vi "Data Format.vi"(9 "Table":refnum<vi>) -> (0 "title":string[](array[string]), 2 "Data":string[](array[string]))   [LabVIEW 2017]
panel:
  out "Error_Description":string
  out "Table":string[][](array[string])
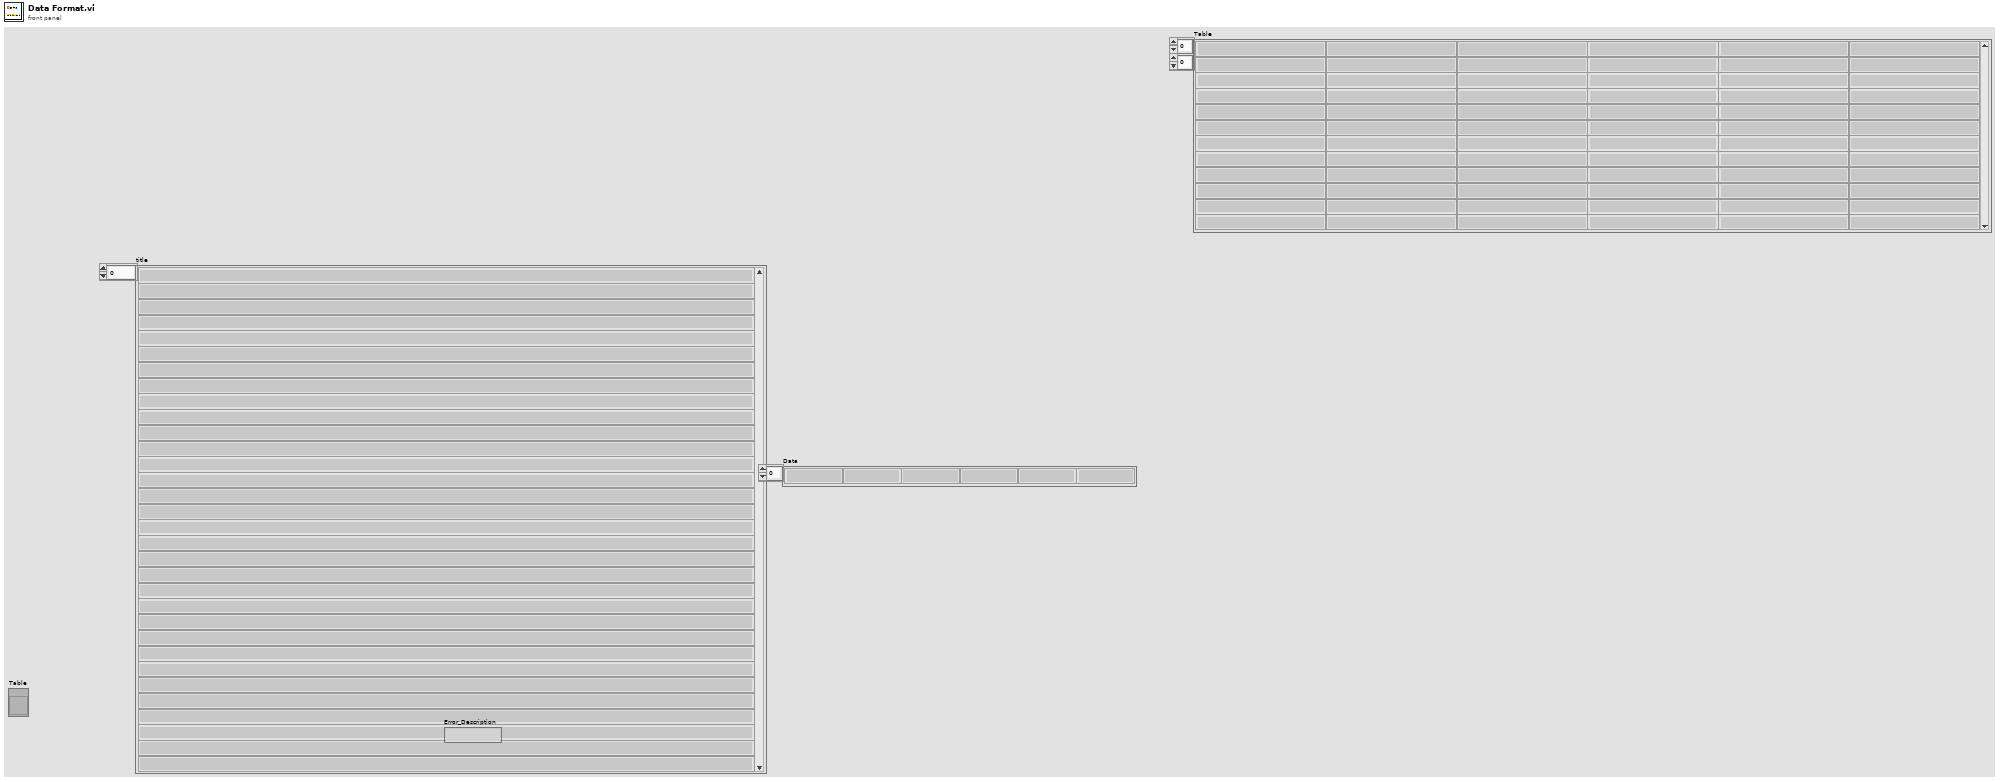
[diagram p1: front panel]
types:
  T1 = typedef "HD Config.ctl" = cluster{" PC":cluster{"PC Address":u8[], "PC Port":i32}, "FCO":cluster{"COM":refnum<visa-resource-name>, "Baudrate":u32}, "DC Power ":cluster{"COM":refnum<visa-resource-name>, "Baudrate":u32}, "PW3336":cluster{"COM":refnum<visa-resource-name>, "Baudrate":u32}, "Lefoo":cluster{"COM":refnum<visa-resource-name>, "Baudrate":u32}, "Tempt&Hum":cluster{"COM":refnum<visa-resource-name>, "Baudrate":u32}, "DIPC":cluster{"COM":refnum<visa-resource-name>}, "Daemon":cluster{"IP Address":string, "Port":u16, "Retry":u16}, "URAT":cluster{"COM":refnum<visa-resource-name>, "Baudrate":u32}, "Fail_resume_mode":bool, "GRR":bool}
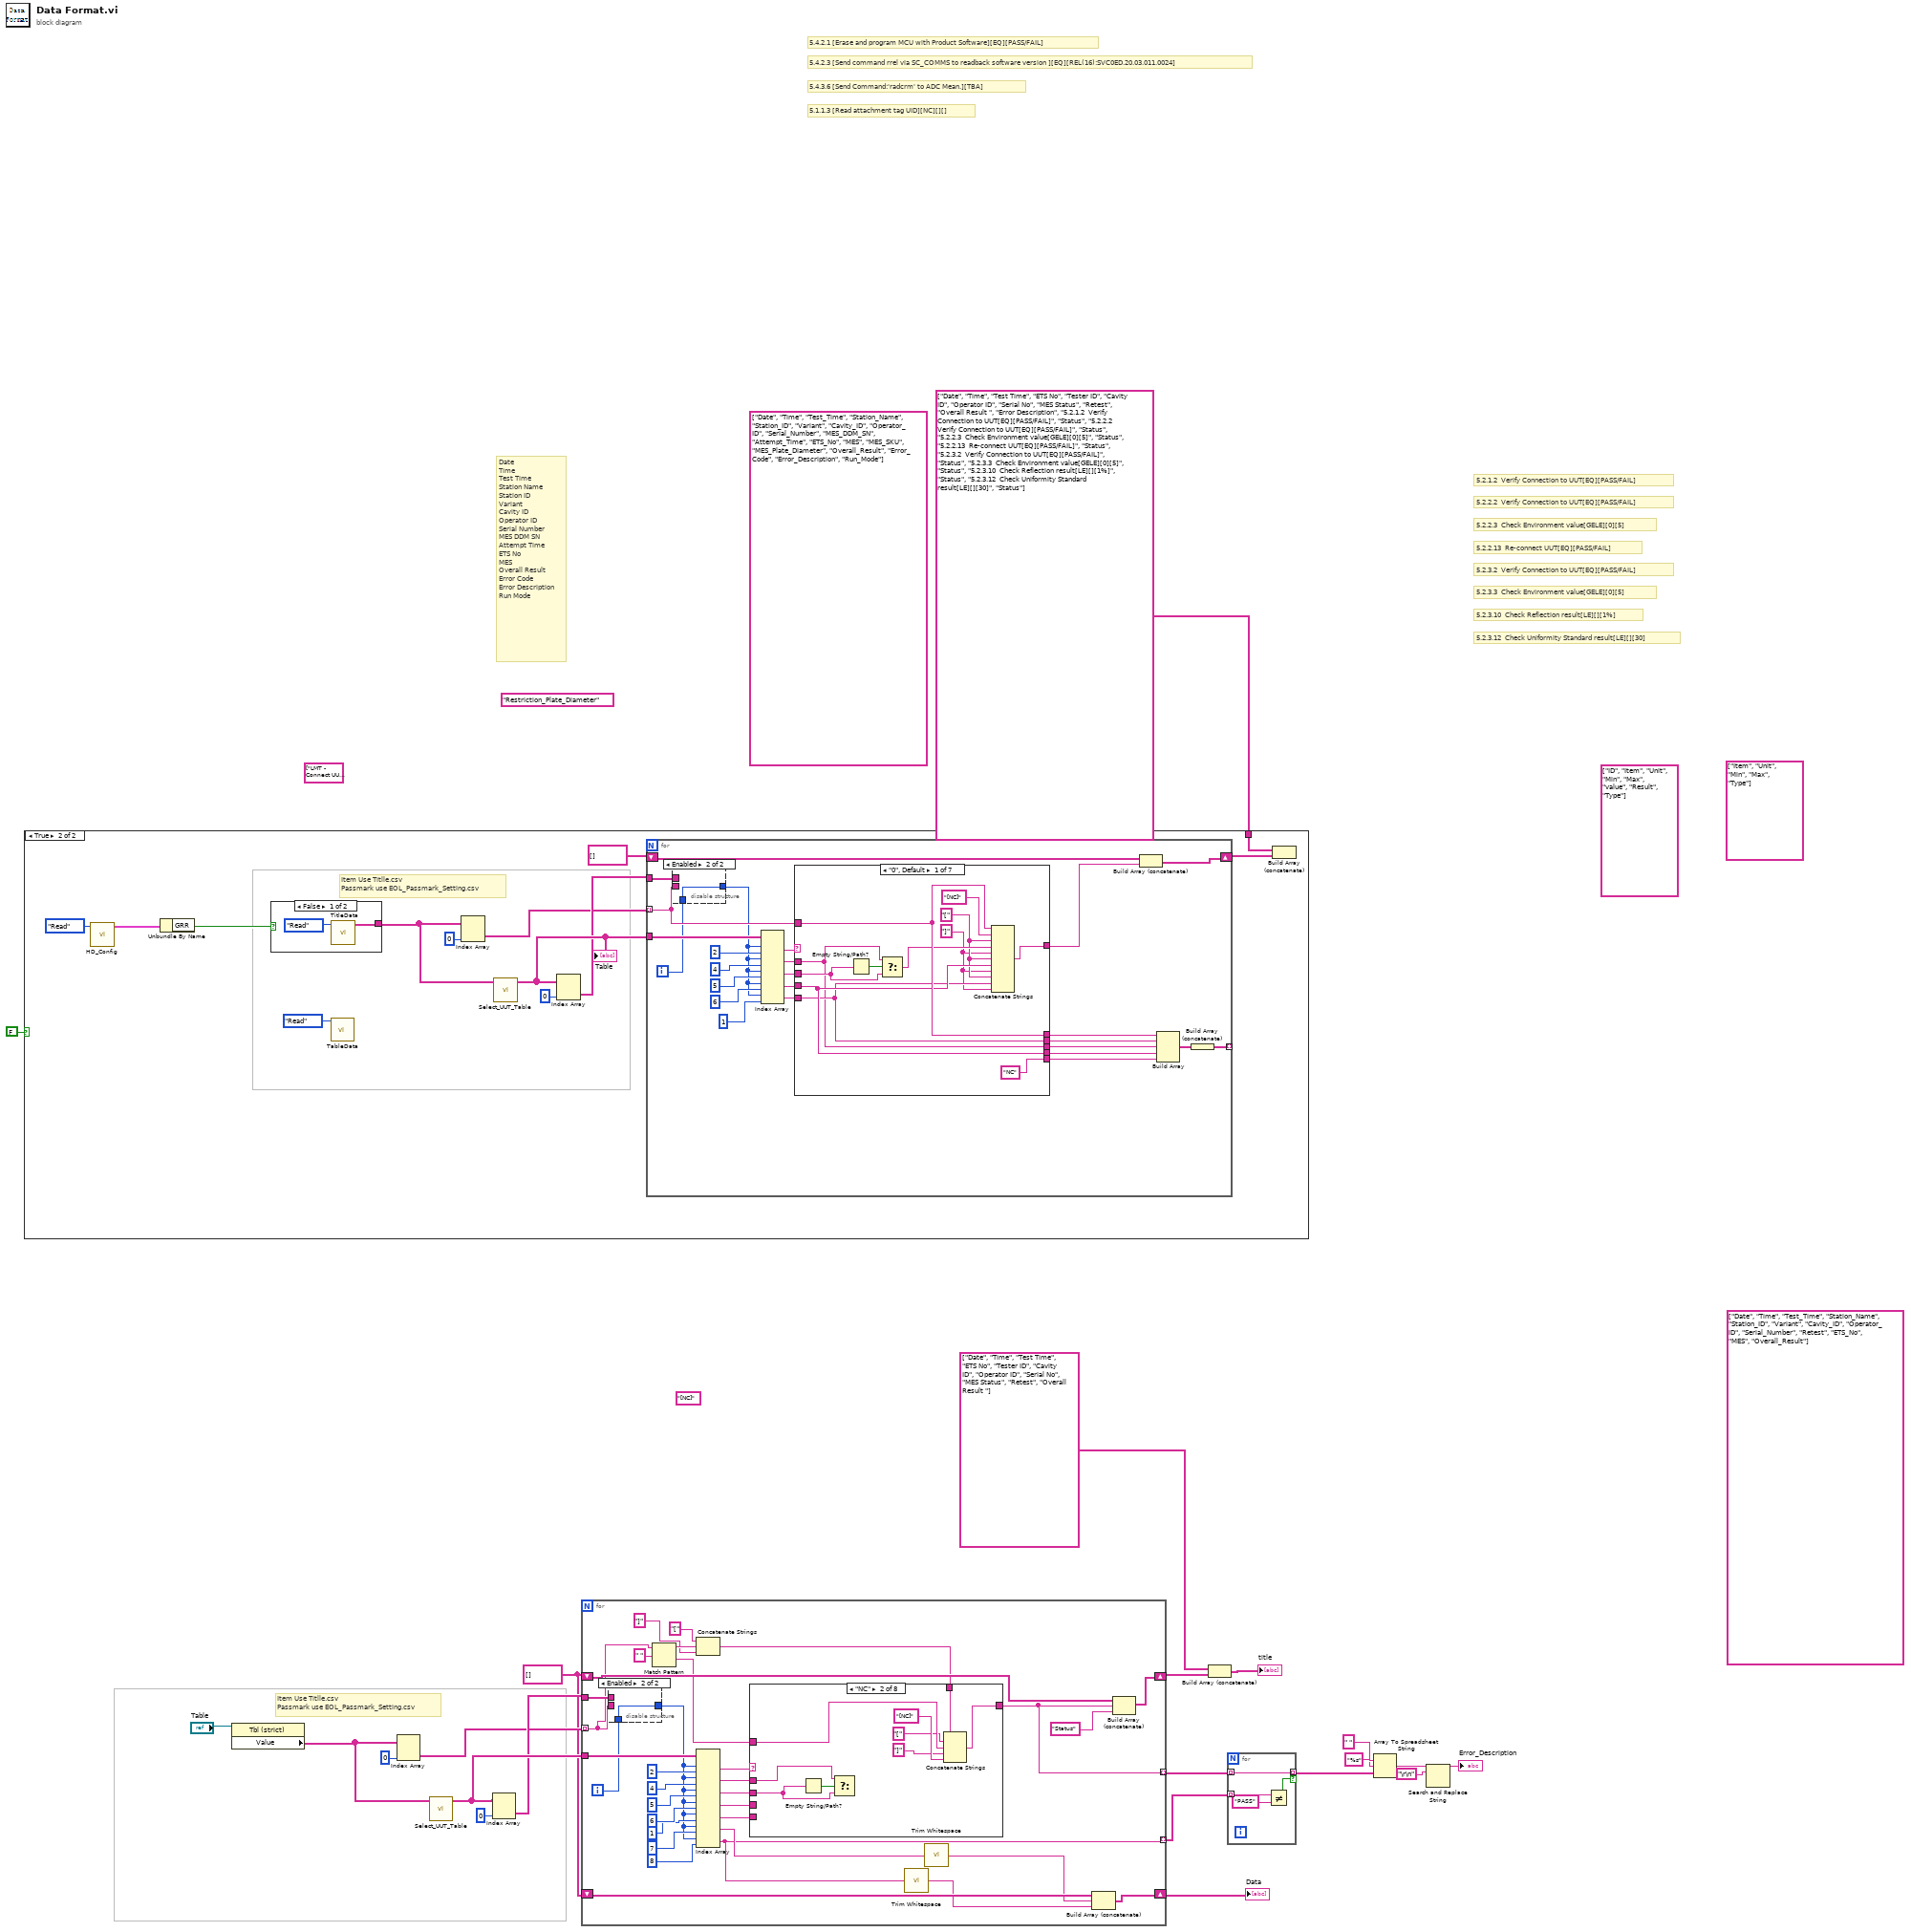
[diagram p0: block diagram]
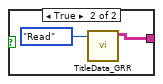
[diagram p3: hidden frame]
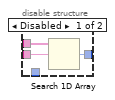
[diagram p4: hidden frame]
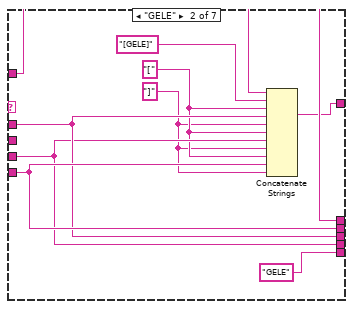
[diagram p5: hidden frame]
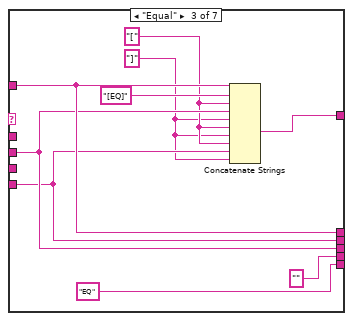
[diagram p6: hidden frame]
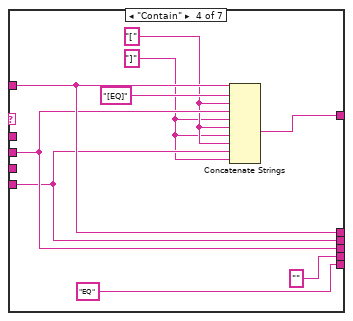
[diagram p7: hidden frame]
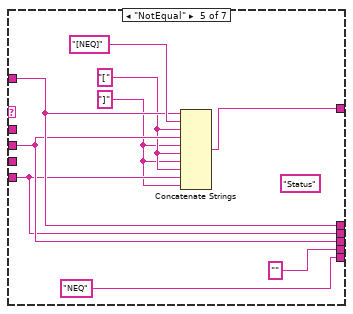
[diagram p8: hidden frame]
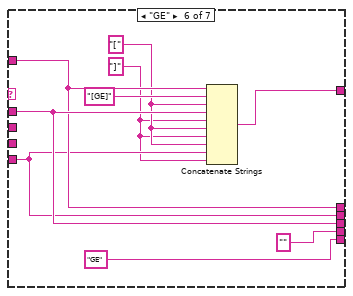
[diagram p9: hidden frame]
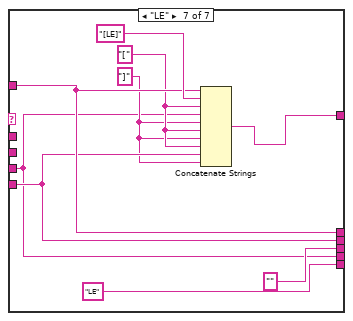
[diagram p10: hidden frame]
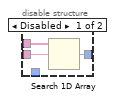
[diagram p11: hidden frame]
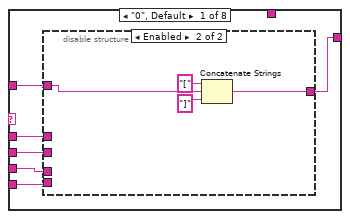
[diagram p12: hidden frame]
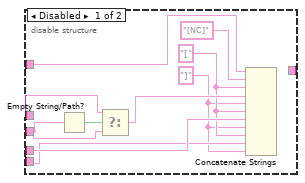
[diagram p13: hidden frame]
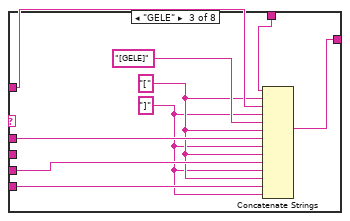
[diagram p14: hidden frame]
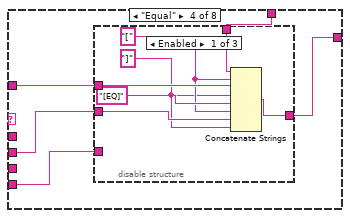
[diagram p15: hidden frame]
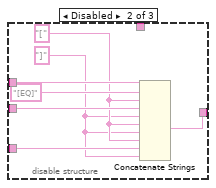
[diagram p16: hidden frame]
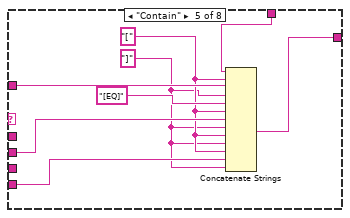
[diagram p18: hidden frame]
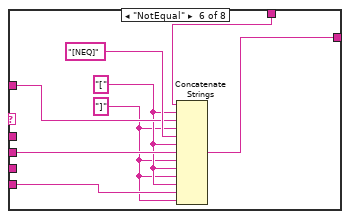
[diagram p19: hidden frame]
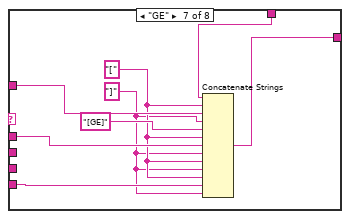
[diagram p20: hidden frame]
diagram:
  (unwired) "[NC]"
  w14 = string[] []
  (unwired) string[] ["Date", "Time", "Test_Time", "Station_Name", "Station_ID", "Variant", "Cavity_ID", "Operator_ID", "Serial_Number", "Retest", "ETS_No", "MES", "Overall_Result"]
  (unwired) "Restriction_Plate_Diameter"
  (unwired) string[] ["ID", "Item", "Unit", "Min", "Max", "value", "Result", "Type"] ("列首字符串[]")
  (unwired) string[] ["LMT - Connect UUT (con COM)", "LMT - Software Version (rrel)", "LMT - Write SKU file (wskuc)", "LMT - SKU file name", "LMT Connect UUT - Error Log", "5.3.2.1 Connect UUT DDM", "Connect UUT DDM - Error Log", "5.3.2.8 Read DDM EOL Timestamp", "5.3.2.8 Read DDM EOL Timestamp - Mode", "5.3.2.8 Read DDM EOL Timestamp - Timestamp", "5.3.2.8 Read DDM EOL Timestamp - Rig ID", "5.3.2.8 Read DDM EOL Timestamp - Passmark ID", "5.3.2.8 Read DDM EOL Timestamp - Passmark Rev", "Read DDM EOL Timestamp - Error Log", "5.3.2.2 Read DDM SW Version before flashing", "5.3.2.2 Software Version before flashing", "Read DDM SW Version before flashing - Error Log", "5.3.2.7 Read Hardware Serial", "Read Hardware Serial - Error Log", "Read DDM SN from UUT", "UUT DDM SN", "Compare Length", "Compare DDM SN with MES SN", "Check DDM SN - Error Log", "5.3.6.2.2 Backup File Data - CAL", "5.3.6.2.2 Backup Data Response - CAL", "5.3.2.3 Flash Firmware Version", "5.3.2.4 Wait Timeout", "5.3.2.5 Check SW Version", "5.3.2.5 Flashing firmware file name", "Flash Firmware Version - Error Log", "5.3.2a.1 Disconnect UUT", "Disconnect UUT - Error Log", "5.3.2a.3 Connect UUT UI", "Connect UUT UI - Error Log", "5.3.2a.4 Flash Firmware Version", "5.3.2a.4 Wait Timeout", "5.3.2a.4 Check SW Version", "5.3.2a.5 Flashing firmware file name", "Flash Firmware Version - Error Log", "5.3.2.6 Read DDM SW Version after flashing", "5.3.2.6 Check DDM SW Version after flashing", "Read DDM SW Version after flashing - Error Log", "5.3.2.10 Set SKU Config Status", "5.3.2.10 Set SKU Config", "5.3.2.10 Set SKU Config File Name", "Set SKU Config - Error Log", "5.3.2.10 Ready Status", "Ready Status - Error Log", "5.3.2.12 Set Device Mode to EOL", "5.3.2.12 DDM EOL mode", "Set Device Mode - Error Log", "5.3.4.34 Wait 1s", "5.3.2.13 DDM Parameter - Voltage", "5.3.2.13 DDM Parameter - Current", "5.3.2.13 DDM Parameter - Power", "5.3.2.13 DDM Parameter - Speed", "5.3.2.13 DDM Parameter - Pressure", "5.3.2.14 Tester Parameter - Voltage", "5.3.2.14 Tester Parameter - Current", "5.3.2.14 Tester Parameter - Power", "5.3.2.14 Tester Parameter - Ambient Pressure", "5.3.2.14 Tester Parameter - Ambient Temperature", "5.3.2.14 Tester Parameter - Pressure Box", "5.3.2.14 Tester Parameter - Reference Ambient Pressure", "5.3.2.15 Calculated Parameter - DDM Pressure Corrected", "5.3.2.15 Calculated Parameter - DDM Real Power", "5.3.2.15 Calculated Parameter - Delta V", "Get and Check Parameter - Error Log", "5.3.3.0 Read BEMF ambient temperature", "5.3.3.0 Calibration Result - eol_cold_bemf_temp", "Read BEMF ambient temperature - Error Log", "5.3.3.0 Set ambient temp to DDM", "5.3.3.0 DDM Ambient Temp", "Set ambient temp to DDM - Error Log", "5.3.4.2 Restriction Plate Diameter", "5.3.4.2 BEMF CAL - Put 13mm Restriction Plate", "Put Restriction Plate - Error Log", "5.3.3.1 Set - Calibrate BEMF both", "5.3.3.1 Get - Calibrate BEMF LSI", "5.3.3.2 Get - Calibration Result - eol_bemf_mp_cold_coef_a", "5.3.3.2 Get - Calibration Result - eol_bemf_mp_cold_coef_b", "5.3.3.2 Get - Calibration Result - eol_bemf_mp_cold_coef_c", "5.3.3.2 Get - Calibration Result - eol_bemf_lsi_cold_ref_coeffs", "5.3.3.2 Get - Calibration Result - eol_bemf_lsi_speed", "5.3.3.2 Get - Calibration Result - eol_bemf_lsi_integral_0", "5.3.3.2 Get - Calibration Result - eol_bemf_lsi_integral_1", "5.3.3.2 Get - Calibration Result - eol_bemf_lsi_integral_2", "5.3.3.2 Get - Calibration Result - eol_cold_bemf", "5.3.3.2 Get - Calibration Result - eol_cold_bemf_fisf", "Get - Calibrate BEMF LSI - Error Log", "5.3.3.3 Finalise Calibration", "5.3.3.4 Wait 1 sec", "Finalise Calibration - Error Log", "5.3.3.1 Get - Calibrate BEMF LSI", "5.3.3.2 Get - Calibration Result - eol_cold_bemf", "5.3.3.2 Get - Calibration Result - eol_cold_bemf_fisf", "5.3.3.2 Compare -Calibration Result - eol_cold_bemf", "5.3.3.2 Compare -Calibration Result - eol_cold_bemf_fisf", "Get & Compare - Calibrate BEMF LSI - Error Log", "5.3.3.3 Reset Power Tune", "5.3.3.4 Reset Power Tune Value", "Reset Power Tune - Error Log", "5.3.3.3 Reset BEMF FISF Calibration", "5.3.3.4 Reset BEMF FISF Calibration Value", "Reset BEMF FISF Calibration - Error Log", "5.3.4.2 ECO - Put 13mm Restriction Plate", "5.3.4.2 Restriction Plate Diameter", "Put Restriction Plate - Error Log", "5.3.4.5 ECO - Motor ON", "5.3.4.5 ECO - Motor ON Mode", "ECO - Motor ON - Error Log", "5.3.4.6 ECO - Motor Speed Stabilisation", "5.3.4.6 ECO - Stabilisation Time", "ECO - Motor Speed Stabilisation - Error Log", "5.3.4.7 ECO - DDM Parameter - Voltage", "5.3.4.7 ECO - DDM Parameter - Current", "5.3.4.7 ECO - DDM Parameter - Power", "5.3.4.7 ECO - DDM Parameter - Measured Power", "5.3.4.7 ECO - DDM Parameter - Speed", "5.3.4.7 ECO - DDM Parameter - Pressure", "5.3.4.7 ECO - DDM Parameter - lsi magnet temp", "5.3.4.7 ECO - DDM Parameter - fisf magnet temp", "5.3.4.7 ECO - DDM Parameter - iir magnet temp", "5.3.4.8 ECO - Tester Parameter - Voltage", "5.3.4.8 ECO - Tester Parameter - Current", "5.3.4.8 ECO - Tester Parameter - Power", "5.3.4.8 ECO - Tester Parameter - Ambient Pressure", "5.3.4.8 ECO - Tester Parameter - Ambient Temperature", "5.3.4.8 ECO - Tester Parameter - Ambient Humidity", "5.3.4.8 ECO - Tester Parameter - Pressure Box", "5.3.4.8 ECO - Tester Parameter - Reference Ambient Pressure", "5.3.4.9 ECO - Calculated Parameter - DDM Pressure Corrected", "5.3.4.9 ECO - Calculated Parameter - DDM Real Power", "5.3.4.9 ECO - Calculated Parameter - Delta V", "5.3.4.9 ECO - Calculated Parameter - Flowrate", "5.3.4.9 ECO - Calculated Parameter - Airwatt", "5.3.4.9 ECO - Formula", "ECO - Get and Check Parameter - Error Log", "PT ECO - Power Tune Mode Status", "PT ECO - Power Tune Set Delta Power Tune", "PT ECO - Power Tune Index", "PT ECO - Power Tune Delta_P", "PT ECO - Power Tune Motor ON Status", "PT ECO - Power Tune Motor ON Mode", "PT ECO - Power Tune Stabilisation Time Status", "PT ECO - Power Tune Stabilisation Delay Time", "PT ECO - DDM Parameter - Voltage", "PT ECO - DDM Parameter - Current", "PT ECO - DDM Parameter - Power", "PT ECO - DDM Parameter - Measured Power", "PT ECO - DDM Parameter - Speed", "PT ECO - DDM Parameter - Pressure", "PT ECO - DDM Parameter - lsi magnet temp", "PT ECO - DDM Parameter - fisf magnet temp", "PT ECO - DDM Parameter - iir magnet temp", "PT ECO - Tester Parameter - Voltage", "PT ECO - Tester Parameter - Current", "PT ECO - Tester Parameter - Power", "PT ECO - Tester Parameter - Ambient Pressure", "PT ECO - Tester Parameter - Ambient Temperature", "PT ECO - Tester Parameter - Ambient Humidity", "PT ECO - Tester Parameter - Pressure Box", "PT ECO - Tester Parameter - Reference Ambient Pressure", "PT ECO - Calculated Parameter - DDM Pressure Corrected", "PT ECO - Calculated Parameter - DDM Real Power", "PT ECO - Calculated Parameter - Delta V", "PT ECO - Calculated Parameter - Flowrate", "PT ECO - Calculated Parameter - Airwatt", "PT ECO - Formula", "PT ECO - Get and Check Parameter - Error Log", "5.3.4.2 BOOST - Put 13mm Restriction Plate", "5.3.4.2 Restriction Plate Diameter", "Put Restriction Plate - Error Log", "5.3.4.5 BOOST - Motor ON", "5.3.4.5 BOOST - Motor ON Mode", "BOOST - Motor ON - Error Log", "5.3.4.6 BOOST - Motor Speed Stabilisation", "5.3.4.6 BOOST - Stabilisation Time", "5.3.4.7 BOOST - DDM Parameter - Voltage", "5.3.4.7 BOOST - DDM Parameter - Current", "5.3.4.7 BOOST - DDM Parameter - Power", "5.3.4.7 BOOST - DDM Parameter - Measured Power", "5.3.4.7 BOOST - DDM Parameter - Speed", "5.3.4.7 BOOST - DDM Parameter - Pressure", "5.3.4.7 BOOST - DDM Parameter - lsi magnet temp", "5.3.4.7 BOOST - DDM Parameter - fisf magnet temp", "5.3.4.7 BOOST - DDM Parameter - iir magnet temp", "5.3.4.8 BOOST - Tester Parameter - Voltage", "5.3.4.8 BOOST - Tester Parameter - Current", "5.3.4.8 BOOST - Tester Parameter - Power", "5.3.4.8 BOOST - Tester Parameter - Ambient Pressure", "5.3.4.8 BOOST - Tester Parameter - Ambient Temperature", "5.3.4.8 BOOST - Tester Parameter - Ambient Humidity", "5.3.4.8 BOOST - Tester Parameter - Pressure Box", "5.3.4.8 BOOST - Tester Parameter - Reference Ambient Pressure", "5.3.4.9 BOOST - Calculated Parameter - DDM Pressure Corrected", "5.3.4.9 BOOST - Calculated Parameter - DDM Real Power", "5.3.4.9 BOOST - Calculated Parameter - Delta V", "5.3.4.9 BOOST - Calculated Parameter - Flowrate", "5.3.4.9 BOOST - Calculated Parameter - Airwatt", "5.3.4.9 BOOST - Formula", "BOOST - Get and Check Parameter - Error Log", "5.3.4.9 BOOST - Check air muscle presence", "5.3.4.9 BOOST - Check air muscle presence Vaule", "BOOST - Check air muscle presence - Error Log", "5.3.4.9 BOOST - Air Muscle Turn Off Status", "5.3.4.9 BOOST - Air Muscle Control", "5.3.3.10 BOOST - Air Muscle Stabilisation Time Status", "5.3.3.10 BOOST - Air Muscle Stabilisation Delay Time", "5.3.4.9 BOOST - Air Muscle Calculated Parameter - Airwatt B", "5.3.4.9 BOOST - Air Muscle Formula", "5.3.4.9 BOOST - Air Muscle Calculate Airwatt Delta", "BOOST - Air Muscle Check - Error Log", "PT BOOST - Power Tune Mode Status", "PT BOOST - Power Tune Set Delta Power Tune", "PT BOOST - Power Tune Index", "PT BOOST - Power Tune Delta_P", "PT BOOST - Power Tune Motor ON Status", "PT BOOST - Power Tune Motor ON Mode", "PT BOOST - Power Tune Stabilisation Time Status", "PT BOOST - Power Tune Stabilisation Delay Time", "PT BOOST - DDM Parameter - Voltage", "PT BOOST - DDM Parameter - Current", "PT BOOST - DDM Parameter - Power", "PT BOOST - DDM Parameter - Measured Power", "PT BOOST - DDM Parameter - Speed", "PT BOOST - DDM Parameter - Pressure", "PT BOOST - DDM Parameter - lsi magnet temp", "PT BOOST - DDM Parameter - fisf magnet temp", "PT BOOST - DDM Parameter - iir magnet temp", "PT BOOST - Tester Parameter - Voltage", "PT BOOST - Tester Parameter - Current", "PT BOOST - Tester Parameter - Power", "PT BOOST - Tester Parameter - Ambient Pressure", "PT BOOST - Tester Parameter - Ambient Temperature", "PT BOOST - Tester Parameter - Ambient Humidity", "PT BOOST - Tester Parameter - Pressure Box", "PT BOOST - Tester Parameter - Reference Ambient Pressure", "PT BOOST - Calculated Parameter - DDM Pressure Corrected", "PT BOOST - Calculated Parameter - DDM Real Power", "PT BOOST - Calculated Parameter - Delta V", "PT BOOST - Calculated Parameter - Flowrate", "PT BOOST - Calculated Parameter - Airwatt", "PT BOOST - Formula", "PT BOOST - Get and Check Parameter - Error Log", "5.3.4.34 Motor OFF", "5.3.4.34 Motor Power", "Motor OFF - Error Log", "5.3.4.34 Wait 1s", "5.3.4.35 Finalise Calibration", "Finalise Calibration - Error Log", "5.3.4.34 ECO - Get AW Calibration Status", "5.3.4.34 ECO - Get AW Calibration value", "5.3.4.34 ECO - Overall Status", "ECO - Get AW Calibration - Error Log", "5.3.4.34 BOOST - Get AW Calibration Status", "5.3.4.34 BOOST - Get AW Calibration value", "5.3.4.34 BOOST - Overall Status", "BOOST - Get AW Calibration - Error Log", "5.3.4.2 MAX - Put 13mm Restriction Plate", "5.3.4.2 Restriction Plate Diameter", "Put Restriction Plate - Error Log", "5.3.4.5 MAX - Motor ON", "5.3.4.5 MAX - Motor ON Mode", "MAX - Motor ON - Error Log", "5.3.4.6 MAX - Motor Speed Stabilisation", "5.3.4.6 MAX - Stabilisation Time", "MAX - Motor Speed Stabilisation - Error Log", "5.3.4.6 Get Average Delta Tmag Status", "5.3.4.6 Get Average Delta Tmag (LSIdelta_FISFdelta_LSItmag_FISFtmag_IIRtmag)", "5.3.4.6 Get Average Delta Tmag LSI", "5.3.4.6 Get Average Delta Tmag FISF", "Get Average Delta Tmag - Error Log", "5.3.4.7 MAX - DDM Parameter - Voltage", "5.3.4.7 MAX - DDM Parameter - Current", "5.3.4.7 MAX - DDM Parameter - Power", "5.3.4.7 MAX - DDM Parameter - Measured Power", "5.3.4.7 MAX - DDM Parameter - Speed", "5.3.4.7 MAX - DDM Parameter - Pressure", "5.3.4.8 MAX - Tester Parameter - Voltage", "5.3.4.8 MAX - Tester Parameter - Current", "5.3.4.8 MAX - Tester Parameter - Power", "5.3.4.8 MAX - Tester Parameter - Ambient Pressure", "5.3.4.8 MAX - Tester Parameter - Ambient Temperature", "5.3.4.8 MAX - Tester Parameter - Ambient Humidity", "5.3.4.8 MAX - Tester Parameter - Pressure Box", "5.3.4.8 MAX - Tester Parameter - Reference Ambient Pressure", "5.3.4.9 MAX - Calculated Parameter - DDM Pressure Corrected", "5.3.4.9 MAX - Calculated Parameter - DDM Real Power", "5.3.4.9 MAX - Calculated Parameter - Delta V", "5.3.4.9 MAX - Calculated Parameter - Flowrate", "5.3.4.9 MAX - Calculated Parameter - Airwatt", "5.3.4.9 MAX - Formula", "MAX - Get and Check Parameter - Error Log", "5.3.3.10 MAX - FISF - Check Average Delta Tmag", "5.3.3.10 MAX - FISF - Check Average Delta Tmag Status", "5.3.3.10 MAX - FISF - BEMF Finetune Result", "BEMF Finetune - Error Log", "MAX tune - Check Airwatts Status", "Calculate Delta Airwatts - MAX tune - Calculate Delta Airwatts", "Calculate Delta Airwatts a - MAX tune - ddm_real_power_a", "Calculate Delta Airwatts b - MAX tune - ddm_real_power_b", "Calculate Delta Airwatts c - MAX tune - Target AW", "Calculate Delta Airwatts d - MAX tune - AW tune extra", "Calculate Delta Airwatts e - MAX tune - Latest AW", "Calculate Delta Airwatts f - MAX tune - correction_factor", "Calculate Delta Airwatts g - MAX tune - P extra", "Calculate Delta Airwatts h - MAX tune - constant power table index", "Calculate Delta Airwatts - MAX tune - Delta P1", "Set AW Tune - MAX tune - Daemon Status", "Set AW Tune - MAX tune - Delta P1 in mW", "Set AW Tune - MAX tune - constant power table index", "Set AW Tune - MAX tune - Drive Mode", "Set AW Tune - MAX tune - Result Airwatt Tune", "5.3.4.5 MAX tune - Motor ON", "5.3.4.5 MAX tune - Motor ON Mode", "5.3.4.6 MAX tune - Motor Speed Stabilisation", "5.3.4.6 MAX tune - Stabilisation Time", "5.3.4.7 MAX tune - DDM Parameter - Voltage", "5.3.4.7 MAX tune - DDM Parameter - Current", "5.3.4.7 MAX tune - DDM Parameter - Power", "5.3.4.7 MAX tune - DDM Parameter - Measured Power", "5.3.4.7 MAX tune - DDM Parameter - Speed", "5.3.4.7 MAX tune - DDM Parameter - Pressure", "5.3.4.7 MAX tune - DDM Parameter - lsi magnet temp", "5.3.4.7 MAX tune - DDM Parameter - fisf magnet temp", "5.3.4.7 MAX tune - DDM Parameter - iir magnet temp", "5.3.4.8 MAX tune - Tester Parameter - Voltage", "5.3.4.8 MAX tune - Tester Parameter - Current", "5.3.4.8 MAX tune - Tester Parameter - Power", "5.3.4.8 MAX tune - Tester Parameter - Ambient Pressure", "5.3.4.8 MAX tune - Tester Parameter - Ambient Temperature", "5.3.4.8 MAX tune - Tester Parameter - Ambient Humidity", "5.3.4.8 MAX tune - Tester Parameter - Pressure Box", "5.3.4.8 MAX tune - Tester Parameter - Reference Ambient Pressure", "5.3.4.9 MAX tune - Calculated Parameter - DDM Pressure Corrected", "5.3.4.9 MAX tune - Calculated Parameter - DDM Real Power", "5.3.4.9 MAX tune - Calculated Parameter - Delta V", "5.3.4.9 MAX tune - Calculated Parameter - Flowrate", "5.3.4.9 MAX tune - Calculated Parameter - Airwatt", "5.3.4.9 MAX tune - Formula", "MAX tune - Get and Check Parameter - Error Log", "MAX finetune - Check Airwatts Status", "Calculate Delta Airwatts - MAX finetune - Calculate Delta Airwatts", "Calculate Delta Airwatts a - MAX finetune - ddm_real_power_a", "Calculate Delta Airwatts b - MAX finetune - ddm_real_power_b", "Calculate Delta Airwatts c - MAX finetune - Target AW", "Calculate Delta Airwatts d - MAX finetune - AW tune extra", "Calculate Delta Airwatts e - MAX finetune - Latest AW", "Calculate Delta Airwatts f - MAX finetune - correction_factor", "Calculate Delta Airwatts g - MAX finetune - P extra", "Calculate Delta Airwatts h - MAX finetune - constant power table index", "Calculate Delta Airwatts - MAX finetune - Delta P2", "Set AW Tune - MAX finetune - Daemon Status", "Set AW Tune - MAX finetune - Delta P2 in mW", "Set AW Tune - MAX finetune - constant power table index", "Set AW Tune - MAX finetune - Drive Mode", "Set AW Tune - MAX finetune - Result Airwatt Finetune", "5.3.4.5 MAX finetune - Motor ON", "5.3.4.5 MAX finetune - Motor ON Mode", "5.3.4.6 MAX finetune - Motor Speed Stabilisation", "5.3.4.6 MAX finetune - Stabilisation Time", "5.3.4.7 MAX finetune - DDM Parameter - Voltage", "5.3.4.7 MAX finetune - DDM Parameter - Current", "5.3.4.7 MAX finetune - DDM Parameter - Power", "5.3.4.7 MAX finetune - DDM Parameter - Measured Power", "5.3.4.7 MAX finetune - DDM Parameter - Speed", "5.3.4.7 MAX finetune - DDM Parameter - Pressure", "5.3.4.7 MAX finetune - DDM Parameter - lsi magnet temp", "5.3.4.7 MAX finetune - DDM Parameter - fisf magnet temp", "5.3.4.7 MAX finetune - DDM Parameter - iir magnet temp", "5.3.4.8 MAX finetune - Tester Parameter - Voltage", "5.3.4.8 MAX finetune - Tester Parameter - Current", "5.3.4.8 MAX finetune - Tester Parameter - Power", "5.3.4.8 MAX finetune - Tester Parameter - Ambient Pressure", "5.3.4.8 MAX finetune - Tester Parameter - Ambient Temperature", "5.3.4.8 MAX finetune - Tester Parameter - Ambient Humidity", "5.3.4.8 MAX finetune - Tester Parameter - Pressure Box", "5.3.4.8 MAX finetune - Tester Parameter - Reference Ambient Pressure", "5.3.4.9 MAX finetune - Calculated Parameter - DDM Pressure Corrected", "5.3.4.9 MAX finetune - Calculated Parameter - DDM Real Power", "5.3.4.9 MAX finetune - Calculated Parameter - Delta V", "5.3.4.9 MAX finetune - Calculated Parameter - Flowrate", "5.3.4.9 MAX finetune - Calculated Parameter - Airwatt", "5.3.4.9 MAX finetune - Formula", "MAX finetune - Get and Check Parameter - Error Log", "5.3.3.10 Check Derate Status", "5.3.3.10 Check Derate Result", "Check Derate Status - Get and Check Parameter - Error Log", "5.3.4.6 Get Delta Tmag After Tuned Status", "5.3.4.6 Delta Tmag FISF", "5.3.4.6 FISF Tmag", "5.3.4.6 IIR Tmag", "Get Delta Tmag After Tuned - Error Log", "5.3.3.10 Get Hot BEMF Status", "5.3.3.10 Get Hot BEMF Result", "Get Hot BEMF Status - Get and Check Parameter - Error Log", "5.3.4.34 Motor OFF", "5.3.4.34 Motor Power", "Motor OFF - Error Log", "5.3.4.34 Wait 1s", "Wait - Error Log", "5.3.3.10 Get DDM Pressure Status", "5.3.3.10 DDM Pressure", "5.3.3.10 Tester Ambient Pressure", "5.3.3.10 Calculate delta Pressure", "Get DDM Pressure Status - Get and Check Parameter - Error Log", "5.3.4.35 Finalise Calibration", "5.3.4.36 Wait 1 sec", "Finalise Calibration - Error Log", "5.3.3.0 Get Cold BEMF Status", "5.3.3.0 Get Cold BEMF - eol_cold_bemf_fisf", "5.3.3.0 Calculate & Check Delta BEMF", "Get Cold BEMF fisf - Error Log", "5.3.4.34 Get AW Calibration Status", "5.3.4.34 Delta P Airwatts Value", "5.3.4.34 Get Airwatts Tune Index 2", "5.3.4.34 Compare Result", "Get AW Calibration - Error Log", "5.3.3.0 Read DDM ambient temperature", "5.3.3.0 Calibration Result - eol_cold_bemf_temp", "Read BEMF ambient temperature - Error Log", "5.3.3.0 Set ambient temp to DDM", "5.3.3.0 DDM Ambient Temp", "Set ambient temp to DDM - Error Log", "5.3.5.1 Reset Task Detect - LL", "5.3.5.1 Reset Task Detect - HL", "5.3.5.1 Reset Task Detect - LH", "5.3.5.1 Reset Task Detect - HH", "5.3.5.1 Reset eol inlet blockage", "5.3.5.2 LL - Put 30mm Restriction Plate", "5.3.5.2 Restriction Plate Diameter", "Put Restriction Plate - Error Log", "5.3.5.4 LL - A2 mode Motor ON", "5.3.5.4 LL - A2 mode Motor Power", "LL -A2 mode Motor ON - Error Log", "5.3.5.5 LL - Motor Speed Stabilisation", "5.3.5.5 LL - Stabilisation Time", "LL - Motor Speed Stabilisation - Error Log", "5.3.5.6 LL - DDM Parameter - Voltage", "5.3.5.6 LL - DDM Parameter - Current", "5.3.5.6 LL - DDM Parameter - Power", "5.3.5.6 LL - DDM Parameter - Measured Power", "5.3.5.6 LL - DDM Parameter - Speed", "5.3.5.6 LL - DDM Parameter - Pressure", "5.3.5.7 LL - Tester Parameter - Voltage", "5.3.5.7 LL - Tester Parameter - Current", "5.3.5.7 LL - Tester Parameter - Power", "5.3.5.7 LL - DDM Real Power", "5.3.5.7 LL - Get and Check Parameter - Error Log", "5.3.5.8 LL - Calibrate Task Detect LL", "5.3.5.8 LL - Set Calibrate Task Detect LL", "5.3.5.8 LL - Calibrate Task Detect - Error Log", "5.3.5.4 HL - BOOST mode Motor ON", "5.3.5.4 HL - BOOST mode Motor Power", "HL - BOOST mode Motor ON - Error Log", "5.3.5.5 HL - Motor Speed Stabilisation", "5.3.5.5 HL - Stabilisation Time", "HL - Motor Speed Stabilisation - Error Log", "5.3.5.6 HL - DDM Parameter - Voltage", "5.3.5.6 HL - DDM Parameter - Current", "5.3.5.6 HL - DDM Parameter - Power", "5.3.5.6 HL - DDM Parameter - Measured Power", "5.3.5.6 HL - DDM Parameter - Speed", "5.3.5.6 HL - DDM Parameter - Pressure", "5.3.5.7 HL - Tester Parameter - Voltage", "5.3.5.7 HL - Tester Parameter - Current", "5.3.5.7 HL - Tester Parameter - Power", "5.3.5.7 HL - DDM Real Power", "5.3.5.7 HL - Get and Check Parameter - Error Log", "5.3.5.8 HL - Calibrate Task Detect HL", "5.3.5.8 HL - Set Calibrate Task Detect HL", "5.3.5.8 HL - Calibrate Task Detect - Error Log", "5.3.5.15 Motor OFF", "5.3.5.15 Motor Power", "Motor OFF - Error Log", "5.3.5.15 Wait 1s", "Wait - Error Log", "5.3.5.2 LH - Put 16mm Restriction Plate", "5.3.5.2 Restriction Plate Diameter", "Put Restriction Plate - Error Log", "5.3.5.4 LH -A2 mode Motor ON", "5.3.5.4 LH - A2 mode Motor Power", "LH - A2 mode Motor ON - Error Log", "5.3.5.5 LH - Motor Speed Stabilisation", "5.3.5.5 LH - Stabilisation Time", "LH - Motor Speed Stabilisation - Error Log", "5.3.5.6 LH - DDM Parameter - Voltage", "5.3.5.6 LH - DDM Parameter - Current", "5.3.5.6 LH - DDM Parameter - Power", "5.3.5.6 LH - DDM Parameter - Measured Power", "5.3.5.6 LH - DDM Parameter - Speed", "5.3.5.6 LH - DDM Parameter - Pressure", "5.3.5.7 LH - Tester Parameter - Voltage", "5.3.5.7 LH - Tester Parameter - Current", "5.3.5.7 LH - Tester Parameter - Power", "5.3.5.7 LH - DDM Real Power", "5.3.5.7 LH - Get and Check Parameter - Error Log", "5.3.5.8 LH - Calibrate Task Detect LH", "5.3.5.8 LH - Set Calibrate Task Detect LH", "5.3.5.8 LH - Calibrate Task Detect - Error Log", "5.3.5.4 HH - BOOST mode Motor ON", "5.3.5.4 HH - BOOST mode Motor Power", "HH - BOOST mode Motor ON - Error Log", "5.3.5.5 HH - Motor Speed Stabilisation", "5.3.5.5 HH - Stabilisation Time", "HH - Motor Speed Stabilisation - Error Log", "5.3.5.6 HH - DDM Parameter - Voltage", "5.3.5.6 HH - DDM Parameter - Current", "5.3.5.6 HH - DDM Parameter - Power", "5.3.5.6 HH - DDM Parameter - Measured Power", "5.3.5.6 HH - DDM Parameter - Speed", "5.3.5.6 HH - DDM Parameter - Pressure", "5.3.5.7 HH - Tester Parameter - Voltage", "5.3.5.7 HH - Tester Parameter - Current", "5.3.5.7 HH - Tester Parameter - Power", "5.3.5.7 HH - DDM Real Power", "5.3.5.7 HH - Get and Check Parameter - Error Log", "5.3.5.8 HH - Calibrate Task Detect HH", "5.3.5.8 HH - Set Calibrate Task Detect HH", "5.3.5.8 HH - Calibrate Task Detect - Error Log", "5.3.5.29 Wait 1s", "Wait - Error Log", "Inlet Blockage Calibration - Motor ON", "Inlet Blockage Calibration - Motor Power", "Inlet Blockage Calibration - Motor ON - Error Log", "Inlet Blockage Calibration - Motor Speed Stabilisation", "Inlet Blockage Calibration - Stabilisation Time", "Inlet Blockage Calibration - Motor Speed Stabilisation - Error Log", "Inlet Blockage Calibration - DDM Parameter - Voltage", "Inlet Blockage Calibration - DDM Parameter - Current", "Inlet Blockage Calibration - DDM Parameter - Power", "Inlet Blockage Calibration - DDM Parameter - Measured Power", "Inlet Blockage Calibration - DDM Parameter - Speed", "Inlet Blockage Calibration - DDM Parameter - Pressure", "Inlet Blockage Calibration - DDM Parameter - lsi magnet temp", "Inlet Blockage Calibration - DDM Parameter - fisf magnet temp", "Inlet Blockage Calibration - DDM Parameter - iir magnet temp", "Inlet Blockage Calibration - Tester Parameter - Voltage", "Inlet Blockage Calibration - Tester Parameter - Current", "Inlet Blockage Calibration - Tester Parameter - Power", "Inlet Blockage Calibration - DDM Real Power", "Inlet Blockage Calibration - Get and Check Parameter - Error Log", "5.3.5.30 Set Calibrate Inlet Blockage", "5.3.5.30 Calibrate Inlet Blockage Value", "5.3.5.31 Calibrate Inlet Blockage - Wait 1s", "Calibrate Inlet Blockage - Error Log", "5.3.5.15 Motor OFF", "5.3.5.15 Motor Power", "Motor OFF - Error Log", "5.3.5.32 Wait 1s", "Wait - Error Log", "5.3.5.35 Get Calibration Inlet Blockage", "5.3.5.35 Calibration Inlet Blockage", "Get Calibration Inlet Blockage - Error Log", "5.3.3.0 Set ambient temp to DDM", "5.3.3.0 DDM Ambient Temp", "Set ambient temp to DDM - Error Log", "5.3.5.33 Finalise Calibration", "5.3.5.34 Wait 1 sec", "Finalise Calibration - Error Log", "5.3.5.35 Get Task Detect LL", "5.3.5.35 Get Task Detect HL", "5.3.5.35 Get Task Detect LH", "5.3.5.35 Get Task Detect HH", "Get Task Detect - Error Log", "5.3.5.35 Get Calibration Inlet Blockage", "5.3.5.35 Calibration Inlet Blockage", "5.3.5.35 Calibration eol cold bemf temp", "5.3.5.35 Compare Task Detect LL", "5.3.5.35 Compare Task Detect HL", "5.3.5.35 Compare Task Detect LH", "5.3.5.35 Compare Task Detect HH", "5.3.5.35 Compare Calibration Inlet Blockage", "5.3.5.35 Compare Calibration eol cold bemf temp", "Compare Task Detect Inlet Blockage - Error Log", "5.3.6.1.2 GOOD UNIT - Clear EEPROM Error Log", "GOOD UNIT - Clear EEPROM Error Log - Error Log", "5.3.6.1.3 GOOD UNIT - Write Product Timestamp", "5.3.6.1.3 GOOD UNIT - Write Product Timestamp - Mode", "5.3.6.1.3 GOOD UNIT - Write Product Timestamp - Timestamp", "5.3.6.1.3 GOOD UNIT - Write Product Timestamp - Rig ID", "5.3.6.1.3 GOOD UNIT - Write Product Timestamp - Passmark ID", "5.3.6.1.3 GOOD UNIT - Write Product Timestamp - Passmark Rev", "GOOD UNIT - Write Product Timestamp - Error Log", "5.3.2.12 GOOD UNIT - Set Device Mode to PROD", "5.3.2.12 GOOD UNIT - DDM PROD mode", "GOOD UNIT - Set Device Mode - Error Log", "5.3.6.1.6 GOOD UNIT - Wait 1s Delay", "GOOD UNIT - Delay - Error Log", "5.3.2.8 GOOD UNIT - Read DDM PROD Timestamp", "5.3.2.8 GOOD UNIT - Read DDM PROD Timestamp - Mode", "5.3.2.8 GOOD UNIT - Read DDM PROD Timestamp - Timestamp", "5.3.2.8 GOOD UNIT - Read DDM PROD Timestamp - Rig ID", "5.3.2.8 GOOD UNIT - Read DDM PROD Timestamp - Passmark ID", "5.3.2.8 GOOD UNIT - Read DDM PROD Timestamp - Passmark Rev", "5.3.2.8 Compare - Read DDM PROD Timestamp", "5.3.2.8 Compare - Read DDM PROD Timestamp - Mode", "5.3.2.8 Compare - Read DDM PROD Timestamp - Timestamp", "5.3.2.8 Compare - Read DDM PROD Timestamp - Rig ID", "5.3.2.8 Compare - Read DDM PROD Timestamp - Passmark ID", "5.3.2.8 Compare - Read DDM PROD Timestamp - Passmark Rev", "GOOD UNIT - Read DDM PROD Timestamp - Error Log", "5.3.6.1.7 GOOD UNIT - Backup File Data", "5.3.6.1.7 GOOD UNIT - Backup File Data  - Error Log", "5.3.2.7 GOOD UNIT - Check Security Bit", "GOOD UNIT - Check Security Bit - Error Log", "5.3.6.1.8 GOOD UNIT - Set Calibration Lock", "GOOD UNIT - Set Calibration Lock - Error Log", "5.3.6.1.9 GOOD UNIT - Disconnect UUT", "GOOD UNIT - Disconnect UUT - Error Log", "5.3.6.2.2 NG UNIT - Read NVM Error", "NG UNIT - Read NVM Error - Error Log", "5.3.2.12 NG UNIT - DDM FCT mode", "5.3.2.12 NG UNIT - DDM FCT mode", "NG UNIT - Set Device Mode - Error Log", "5.3.6.2.2 NG UNIT - Backup File Data - CAL", "5.3.6.2.2 NG UNIT - Backup File Data - ERROR", "5.3.6.2.2 NG UNIT - Backup File Data - USAGE", "NG UNIT - Backup File Data - Error Log", "5.3.6.2.4 NG UNIT - Disconnect UUT", "NG UNIT - Disconnect UUT - Error Log"] ("数组 2")
  (unwired) string[] ["Item", "Unit", "Min", "Max", "Type"] ("列首字符串[]")
  (unwired) string[] ["Date", "Time", "Test_Time", "Station_Name", "Station_ID", "Variant", "Cavity_ID", "Operator_ID", "Serial_Number", "MES_DDM_SN", "Attempt_Time", "ETS_No", "MES", "MES_SKU", "MES_Plate_Diameter", "Overall_Result", "Error_Code", "Error_Description", "Run_Mode"]
  # "Item Use Titlle.csv\nPassmark use EOL_Passmark_Setting.csv"
  # "5.2.3.12  Check Uniformity Standard result[LE][][30]"
  # "5.2.3.10  Check Reflection result[LE][][1%]"
  # "5.2.3.3  Check Environment value[GELE][0][5]"
  # "5.2.3.2  Verify Connection to UUT[EQ][PASS/FAIL]"
  # "5.2.2.13  Re-connect UUT[EQ][PASS/FAIL]"
  # "5.2.2.3  Check Environment value[GELE][0][5]"
  # "5.2.2.2  Verify Connection to UUT[EQ][PASS/FAIL]"
  # "5.2.1.2  Verify Connection to UUT[EQ][PASS/FAIL]"
  # "5.4.3.6 [Send Command:'radcrm' to ADC Mean.][TBA]"
  # "5.4.2.3 [Send command rrel via SC_COMMS to readback software version ][EQ][REL(16):SVC0ED.20.03.011.0024]"
  # "5.4.2.1 [Erase and program MCU with Product Software][EQ][PASS/FAIL]"
  # "5.1.1.3 [Read attachment tag UID][NC][][]"
  # "Date\nTime\nTest Time\nStation Name\nStation ID\nVariant\nCavity ID\nOperator ID\nSerial Number\nMES DDM SN\nAttempt Time\nETS No\nMES\nOverall Result\nError Code\nError Description\nRun Mode"
  n1 = case shown="True" FALSE {
    tunnel: string[] ["Date", "Time", "Test Time", "ETS No", "Tester ID", "Cavity ID", "Operator ID", "Serial No", "MES Status", "Retest", "Overall Result ", "Error Description", "5.2.1.2  Verify Connection to UUT[EQ][PASS/FAIL]", "Status", "5.2.2.2  Verify Connection to UUT[EQ][PASS/FAIL]", "Status", "5.2.2.3  Check Environment value[GELE][0][5]", "Status", "5.2.2.13  Re-connect UUT[EQ][PASS/FAIL]", "Status", "5.2.3.2  Verify Connection to UUT[EQ][PASS/FAIL]", "Status", "5.2.3.3  Check Environment value[GELE][0][5]", "Status", "5.2.3.10  Check Reflection result[LE][][1%]", "Status", "5.2.3.12  Check Uniformity Standard result[LE][][30]", "Status"] ("title") -> [_ w23]
    frame False {
    }
    frame True {
      # "Item Use Titlle.csv\nPassmark use EOL_Passmark_Setting.csv"
      n2 = call "HD_Config.vi"("Step"=enum16{"Initial", "Write", "Read"}."Read") -> ("HD Config out"=w25:T1)  [unwired: 9 in, 1 out]
      n3 = Unbundle By Name(w25) -> ("GRR"=w24:bool)
      n4 = case shown="False" w24 {
        tunnel: [w36 w38] -> w28
        frame False {
          n5 = call "TitleData.vi"("Step"=enum16{"Initial", "Write", "Read"}."Read") -> ("Tabledata Out"=w36:string[][])  [unwired: 9 in, 1 out]
        }
        frame True {
          n6 = call "TitleData_GRR.vi"("Step"=enum16{"Initial", "Write", "Read"}."Read") -> ("Tabledata Out"=w38:string[][])  [unwired: 9 in, 1 out]
        }
      }
      n7 = call "TableData.vi"("Step"=enum16{"Initial", "Write", "Read"}."Read") -> ()  [unwired: 9 in, 2 out]
      n8 = Index Array "Index Array"(array=w28, index (col)=0 ("禁用的索引 (列)")) -> (element=w29:string[])  [unwired: 1 in]
      n9 = call "Select_UUT_Table.vi"("all Table"=w28) -> ("Table"=w35:string[][])  [unwired: 9 in, 1 out]
      "Table" <- w35
      n10 = Index Array(array=w35, index (col)=0 ("禁用的索引 (列)")) -> (element=w33:string[])  [unwired: 1 in]
      n11 = for {
        tunnel: w29 -> [w52] mode=indexing
        tunnel: w35 -> [w63]
        tunnel: w33 -> [w64]
        shift-right: [w53] -> w31
        shift-left: string[] [] -> [w54]
        tunnel: [w45] -> _ mode=indexing
        i -> [w40]
        n12 = disable-structure shown="Enabled" {
          disable-tunnel: w64 -> [w67 _]
          disable-tunnel: w52 -> [w66 _]
          disable-tunnel: [w65 w68] -> w42
          disable-tunnel: w40 -> [_ w68]
          frame Disabled {
            n13 = Search 1D Array(1D array=w67, element=w66) -> (index of element=w65:i32)  [unwired: 1 in]
          }
          frame Enabled {
          }
        }
        n14 = Index Array(array=w63, index (row) #1=w42, index (col) #1=2 ("禁用的索引 (列)"), index (row) #2=w42, index (col) #2=4 ("禁用的索引 (列)"), index (row) #3=w42, index (col) #3=5 ("禁用的索引 (列)"), index (row) #4=w42, index (col) #4=6 ("禁用的索引 (列)"), index (row) #5=w42, index (col) #5=1 ("索引 (列)")) -> (element #1=w61:string, element #2=w57:string, element #3=w56:string, element #4=w55:string, element #5=w43:string)
        n15 = case shown="\"0\", Default" w61 {
          tunnel: w57 -> [w72 w84 _ _ _ w124 _]
          tunnel: w56 -> [w73 _ w95 w104 w113 _ _]
          tunnel: w55 -> [w76 w83 _ _ _ _ w126]
          tunnel: [w77 w86 w93 w102 w111 w120 w130] -> w41
          tunnel: w52 -> [w79 w88 w97 w106 w115 w123 w133]
          tunnel: [w79 w88 w97 w106 w115 w123 w133] -> w51
          tunnel: [w72 w84 w95 w104 w113 w124 "" ("String")] -> w50
          tunnel: [w76 w83 "" ("String") "" ("String") "" ("String") "" ("String") w126] -> w49
          tunnel: ["NC" "GELE" "EQ" "EQ" "NEQ" "GE" "LE"] -> w48
          tunnel: [w75 w85 w92 w101 w109 w119 w129] -> w46
          tunnel: w43 -> [w75 w85 w92 w101 w109 w119 w129]
          frame "0", Default {
            w69 = "]" ("字符串")
            w70 = "[" ("字符串")
            n16 = Empty String/Path?(string/path=w73) -> (empty?=w74:bool)
            n17 = Select(t=w72, s=w74, f=w73) -> (s? t:f=w71:string)
            n18 = Concatenate Strings(w79, "[NC]", w70, w71, w69, w70, w76, w69, w70, w75, w69) -> (w77:string)
          }
          frame "GELE" {
            w81 = "]" ("字符串")
            w82 = "[" ("字符串")
            n19 = Concatenate Strings(w88, "[GELE]", w82, w84, w81, w82, w83, w81, w82, w85, w81) -> (w86:string)
          }
          frame "Equal" {
            w90 = "]" ("字符串")
            w91 = "[" ("字符串")
            n20 = Concatenate Strings(w97, "[EQ]", w91, w95, w90, w91, w90, w91, w92, w90) -> (w93:string)
          }
          frame "Contain" {
            w99 = "]" ("字符串")
            w100 = "[" ("字符串")
            n21 = Concatenate Strings(w106, "[EQ]", w100, w104, w99, w100, w99, w100, w101, w99) -> (w102:string)
          }
          frame "NotEqual" {
            (unwired) "Status" ("元素")
            w108 = "]" ("字符串")
            w110 = "[" ("字符串")
            n22 = Concatenate Strings(w115, "[NEQ]", w110, w113, w108, w110, w108, w110, w109, w108) -> (w111:string)
          }
          frame "GE" {
            w117 = "]" ("字符串")
            w118 = "[" ("字符串")
            n23 = Concatenate Strings(w123, "[GE]", w118, w124, w117, w118, w117, w118, w119, w117) -> (w120:string)
          }
          frame "LE" {
            w127 = "]" ("字符串")
            w128 = "[" ("字符串")
            n24 = Concatenate Strings(w133, "[LE]", w128, w126, w127, w128, w127, w128, w129, w127) -> (w130:string)
          }
        }
        n25 = Build Array (concatenate)(w54, w41) -> (w53:string[])
        n26 = Build Array ("创建数组")(w51, w46, w50, w49, w48) -> (w47:string[])
        n27 = Build Array (concatenate) ("创建数组")(w47) -> (w45:string[])
      }
      n28 = Build Array (concatenate)(w23, w31) -> ()  [unwired: 1 out]
    }
  }
  n29 = property class="Tbl (strict)"(reference="Table") -> ("Value"=w15:string[][])  [unwired: 1 in, 2 out]
  n30 = Index Array "Index Array"(array=w15, index (col)=0 ("禁用的索引 (列)")) -> (element=w17:string[])  [unwired: 1 in]
  n31 = call "Select_UUT_Table.vi"("all Table"=w15) -> ("Table"=w22:string[][])  [unwired: 9 in, 1 out]
  n32 = Index Array(array=w22, index (col)=0 ("禁用的索引 (列)")) -> (element=w20:string[])  [unwired: 1 in]
  n33 = for {
    tunnel: w17 -> [w142] mode=indexing
    tunnel: w22 -> [w166]
    tunnel: w20 -> [w167]
    shift-right: [w156] -> w19
    shift-left: w14 -> [w157]
    shift-right: [w149] -> w13
    shift-left: w14 -> [w150]
    tunnel: [w146] -> w12 mode=indexing
    tunnel: [w136] -> w11 mode=indexing
    i -> [w153]
    n34 = disable-structure shown="Enabled" {
      disable-tunnel: w167 -> [w170 _]
      disable-tunnel: w142 -> [w169 _]
      disable-tunnel: [w168 w171] -> w148
      disable-tunnel: w153 -> [_ w171]
      frame Disabled {
        n35 = Search 1D Array(1D array=w170, element=w169) -> (index of element=w168:i32)  [unwired: 1 in]
      }
      frame Enabled {
      }
    }
    n36 = Match Pattern(string=w142, regular expression=" ") -> (before substring=w145:string, after substring=w141:string)  [unwired: 1 in, 2 out]
    n37 = Concatenate Strings("[" ("字符串"), w145, "]" ("字符串")) -> (w140:string)
    n38 = Index Array(array=w166, index (row) #1=w148, index (col) #1=2 ("禁用的索引 (列)"), index (row) #2=w148, index (col) #2=4 ("禁用的索引 (列)"), index (row) #3=w148, index (col) #3=5 ("禁用的索引 (列)"), index (row) #4=w148, index (col) #4=6 ("禁用的索引 (列)"), index (row) #5=w148, index (col) #5=1 ("索引 (列)"), index (row) #6=w148, index (col) #6=7 ("disabled index (col)"), index (row) #7=w148, index (col) #7=8 ("disabled index (col)")) -> (element #1=w164:string, element #2=w160:string, element #3=w159:string, element #4=w158:string, element #5=w154:string, element #6=w138:string, element #7=w136:string)
    n39 = case shown="\"NC\"" w164 {
      tunnel: w160 -> [w174 w195 w205 _ _ _ w251 _]
      tunnel: w159 -> [w175 w196 _ w213 w234 w242 _ _]
      tunnel: w158 -> [w177 _ w204 _ _ _ _ w256]
      tunnel: [w172 w198 w207 w212 w233 w241 w249 w258] -> w146
      tunnel: w141 -> [w173 w199 w208 w214 w235 w243 w250 w259]
      tunnel: w154 -> [w176 _ w206 w211 w232 w240 w248 w257]
      tunnel: w140 -> [_ w192 w201 w210 w229 w237 w245 w253]
      frame "0", Default {
        n40 = disable-structure shown="Enabled" {
          disable-tunnel: w177 -> [w186 _]
          disable-tunnel: w176 -> [w185 _]
          disable-tunnel: w175 -> [w183 _]
          disable-tunnel: w174 -> [w182 _]
          disable-tunnel: w173 -> [w178 w191]
          disable-tunnel: [_ w190] -> w172
          frame Disabled {
            w179 = "]" ("字符串")
            w180 = "[" ("字符串")
            n41 = Empty String/Path?(string/path=w183) -> (empty?=w184:bool)
            n42 = Select(t=w182, s=w184, f=w183) -> (s? t:f=w181:string)
            n43 = Concatenate Strings(w178, "[NC]", w180, w181, w179, w180, w186, w179, w180, w185, w179) -> ()  [unwired: 1 out]
          }
          frame Enabled {
            n44 = Concatenate Strings("[" ("string"), w191, "]" ("string")) -> (w190:string)
          }
        }
      }
      frame "NC" {
        n45 = Empty String/Path?(string/path=w196) -> (empty?=w197:bool)
        n46 = Select(t=w195, s=w197, f=w196) -> ()  [unwired: 1 out]
        n47 = Concatenate Strings(w192, "[" ("字符串"), w199, "]" ("字符串"), "[NC]") -> (w198:string)
      }
      frame "GELE" {
        w202 = "]" ("字符串")
        w203 = "[" ("字符串")
        n48 = Concatenate Strings(w201, w203, w208, w202, "[GELE]", w203, w205, w202, w203, w204, w202, w203, w206, w202) -> (w207:string)
      }
      frame "Equal" {
        n49 = disable-structure shown="Enabled" {
          disable-tunnel: w214 -> [w220 w227 _]
          disable-tunnel: w213 -> [w219 w226 _]
          disable-tunnel: [w218 w225 _] -> w212
          disable-tunnel: w211 -> [_ w224 _]
          disable-tunnel: w210 -> [w215 _ _]
          frame Enabled {
            w216 = "]" ("字符串")
            w217 = "[" ("字符串")
            n50 = Concatenate Strings(w215, w217, w220, w216, "[EQ]", w217, w219, w216) -> (w218:string)
          }
          frame Disabled {
            w222 = "]" ("字符串")
            w223 = "[" ("字符串")
            n51 = Concatenate Strings(w227, "[EQ]", w223, w226, w222, w223, w222, w223, w224, w222) -> (w225:string)
          }
          frame Disabled {
          }
        }
      }
      frame "Contain" {
        w230 = "]" ("字符串")
        w231 = "[" ("字符串")
        n52 = Concatenate Strings(w229, w231, w235, w230, "[EQ]", w231, w234, w230, w231, w230, w231, w232, w230) -> (w233:string)
      }
      frame "NotEqual" {
        w238 = "]" ("字符串")
        w239 = "[" ("字符串")
        n53 = Concatenate Strings(w237, w239, w243, w238, "[NEQ]", w239, w242, w238, w239, w238, w239, w240, w238) -> (w241:string)
      }
      frame "GE" {
        w246 = "]" ("字符串")
        w247 = "[" ("字符串")
        n54 = Concatenate Strings(w245, w247, w250, w246, "[GE]", w247, w251, w246, w247, w246, w247, w248, w246) -> (w249:string)
      }
      frame "LE" {
        w254 = "]" ("字符串")
        w255 = "[" ("字符串")
        n55 = Concatenate Strings(w253, w255, w259, w254, "[LE]", w255, w256, w254, w255, w254, w255, w257, w254) -> (w258:string)
      }
    }
    n56 = call <vilib>:"Trim Whitespace.vi"("string"=w136) -> ("trimmed string"=w135:string)  [unwired: 1 in]
    n57 = call <vilib>:"Trim Whitespace.vi"("string"=w138) -> ("trimmed string"=w137:string)  [unwired: 1 in]
    n58 = Build Array (concatenate)(w150, w137, w135) -> (w149:string[])
    n59 = Build Array (concatenate)(w157, w146, "Status" ("element")) -> (w156:string[])
  }
  "Data" <- w13
  n60 = Build Array (concatenate)(string[] ["Date", "Time", "Test Time", "ETS No", "Tester ID", "Cavity ID", "Operator ID", "Serial No", "MES Status", "Retest", "Overall Result "] ("title_beforedata"), w19) -> (→"title":string[])
  n61 = for {
    tunnel: [w264] -> w6 mode=indexing if=w261
    tunnel: w12 -> [w264] mode=indexing
    tunnel: w11 -> [w263] mode=indexing
    n62 = Not Equal?(x=w263, y="PASS") -> (x != y?=w261:bool)
  }
  n63 = Array To Spreadsheet String(delimiter (Tab)=" ", array=w6, 3:"%s" ("delimiter (Tab)")) -> (spreadsheet string=w8:string)
  n64 = Search and Replace String(input string=w8, search string="\r\n") -> (result string=→"Error_Description":string)  [unwired: 6 in, 3 out]
